vi "List COM port.vi"(8 "error in (no error)":errorcluster) -> (0 "error out":errorcluster, 3 "COM Ports":string[](array[string]))   [LabVIEW 2018, in "Thorlabs_FW102C.lvlib"]
doc: "Establishes communication with the instrument and optionally performs an instrument identification query and/or an instrument reset. It also places the instrument in a default state needed for other instrument driver operations. Therefore, call this VI before calling other instrument driver VIs for this instrument. Generally, you need to call the Initialize VI only once at the beginning of an application."
uses:
  Thorlabs_FW102C.lvlib
  <instrlib>/Thorlabs_FW102C/Library/FilterWheel102_win32.dll
  Library/FilterWheel102_win64.dll
panel:
  out "return type":i32
  # "(c) 2015 <Thorlabs>.  ALL RIGHTS RESERVED."
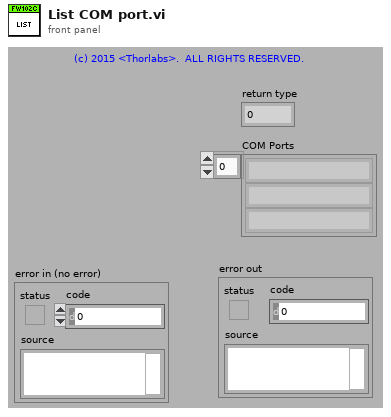
[diagram p1: front panel]
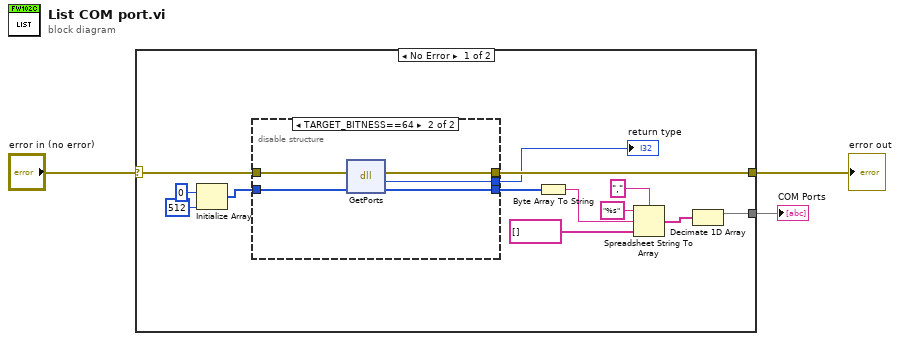
[diagram p0: block diagram]
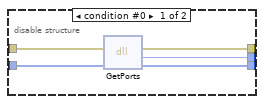
[diagram p2: hidden frame]
diagram:
  n1 = case shown="No Error" "error in (no error)" {
    selector: "error in (no error)" -> [w16 w27]
    tunnel: [w15 w27] -> w3
    tunnel: [w10 _] -> w1
    frame No Error {
      n2 = Initialize Array(u8 0 ("element"), 512 ("dimension size")) -> (w6:u8[])
      n3 = disable-structure shown="TARGET_BITNESS==64" {
        disable-tunnel: w16 -> [w21 w26]
        disable-tunnel: [w20 w25] -> w15
        disable-tunnel: [w19 w23] -> w9
        disable-tunnel: w6 -> [w18 w24]
        disable-tunnel: [w17 w22] -> w4
        frame condition #0 {
          n4 = dll-call lib="E:/Program Files (x86)/National Instruments/LabVIEW 2011/instr.lib/Thorlabs_FW102C/Library/FilterWheel102_win32.dll" fn="GetPorts"(error in=w21, "ports"=w18) -> (error out=w20:errorcluster, "return type"=w17:i32, "ports"=w19:u8[])  [unwired: 2 in, 1 out]
        }
        frame condition #1 (active) {
          n5 = dll-call lib="C:/Users/astrolab/Desktop/Labview_code/Thorlabs_FW102C/Library/FilterWheel102_win64.dll" fn="GetPorts"(error in=w26, "ports"=w24) -> (error out=w25:errorcluster, "return type"=w22:i32, "ports"=w23:u8[])  [unwired: 2 in, 1 out]
        }
      }
      "return type" <- w4
      n6 = Byte Array To String(unsigned byte array=w9) -> (string=w5:string)
      n7 = Spreadsheet String To Array(delimiter (Tab)=",", format string="%s", spreadsheet string=w5, array type (2D Dbl)=string[] []) -> (array=w11:string[])
      n8 = Decimate 1D Array(w11) -> (w10:string[])  [unwired: 1 out]
    }
    frame Error {
    }
  }
  "error out" <- w3
  "COM Ports" <- w1
